vi "DataLog Log String_srv.vi"(0 "tag":string, 5 "string":string, 7 "certificate":string, 9 "database (current)":string) -> (15 "error out":errorcluster)   [LabVIEW 2012]
uses:
  clientsrv/typedefs/t_ClientSrv Access Levels.ctl
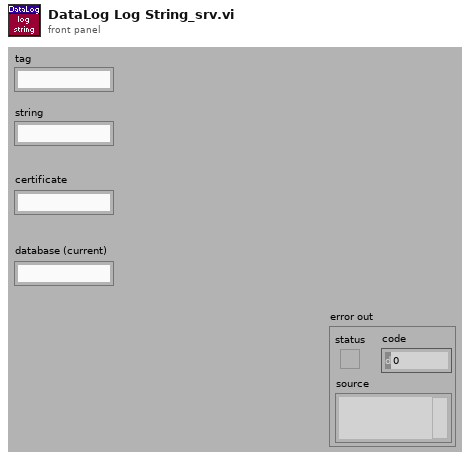
[diagram p1: front panel]
types:
  T1 = typedef "t_ClientSrv Access Levels.ctl" = enum16{"observer", "operator", "local"}
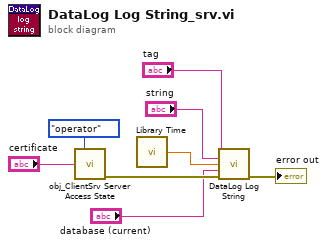
[diagram p0: block diagram]
diagram:
  n1 = call "obj_ClientSrv Server Access State.vi"("access level"=t_ClientSrv_Access_Levels."operator", "certificate in"="certificate") -> ("error out"=w6:errorcluster)  [unwired: 11 in, 2 out]
  n2 = call "Library Time.vi"() -> ("time"=w1:dbl)  [unwired: 1 in]
  n3 = call "DataLog Log String.vi"("tag"="tag", "string"="string", "time"=w1, "database (current)"="database (current)", "error in (no error)"=w6) -> ("error out"=→"error out":errorcluster)  [unwired: 10 in]
